vi "Get Wiimote.vi"(8 "error in (no error)":errorcluster, 9 "Wiimote Player #":i32, 11 "LV Wiimote Interface in":T1) -> (0 "error out":errorcluster, 2 "Wiimote":refnum<k24>, 3 "LV Wiimote Interface out":T1)   [LabVIEW 2012, in "LV Wiimote Interface.lvclass"]
uses:
  LV Wiimote Interface.lvclass
  Controls/LV Wiimote Interface.ctl
  C:/Program Files/National Instruments/LabVIEW 2012/vi.lib/LabVIEW Hacker/WiiMote/Dependencies/WiimoteLib.dll
  Program Files/National Instruments/LabVIEW 2012/vi.lib/LabVIEW Hacker/WiiMote/Dependencies/WiimoteLib.dll
  LV Wiimote Interface.lvclass/LV Wiimote Interface.ctl
  <vilib>/Utility/error.llb/Error Cluster From Error Code.vi
  <vilib>/ErrorRing/Error Ring.xnode
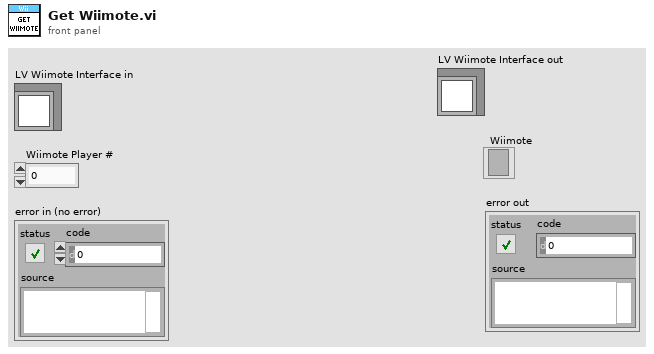
[diagram p1: front panel]
types:
  T1 = typedef "LV Wiimote Interface.ctl" = refnum<class "LV Wiimote Interface.lvclass">
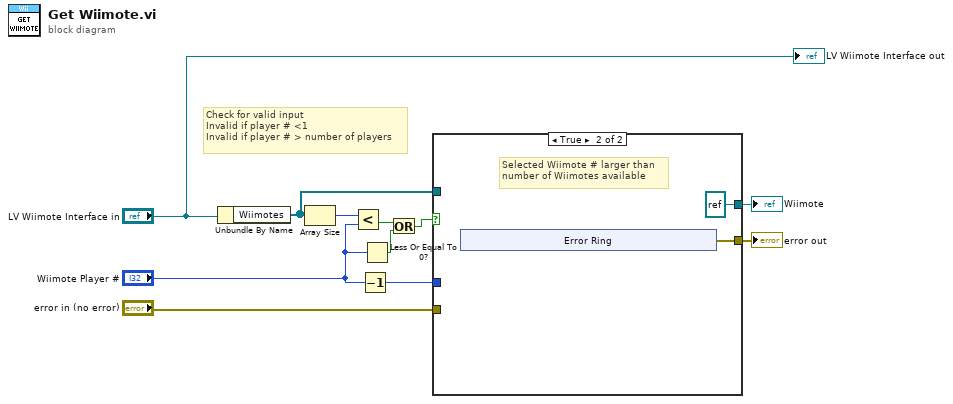
[diagram p0: block diagram]
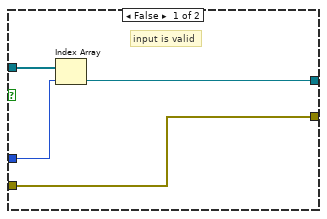
[diagram p2: hidden frame]
diagram:
  # "Check for valid input\nInvalid if player # <1\nInvalid if player # > number of players"
  n1 = Unbundle By Name("LV Wiimote Interface in") -> ("Wiimotes"=w10:refnum<k24>[])
  n2 = Array Size(array=w10) -> (size(s)=w11:i32)
  n3 = Less?(x=w11, y="Wiimote Player #") -> (x < y?=w3:bool)
  n4 = Decrement(x="Wiimote Player #") -> (x-1=w5:i32)
  n5 = Less Or Equal To 0?(x="Wiimote Player #") -> (x <= 0?=w2:bool)
  n6 = Or(x=w3, y=w2) -> (x .or. y?=w1:bool)
  n7 = case shown="True" w1 {
    tunnel: w10 -> [w15 _]
    tunnel: "error in (no error)" -> [w13 _]
    tunnel: [w13 w17] -> w8
    tunnel: [w14 refnum<k24> refnum ("Wiimote")] -> w7
    tunnel: w5 -> [w12 _]
    frame False {
      # "input is valid"
      n8 = Index Array(array=w15, index=w12) -> (element=w14:refnum<k24>)
    }
    frame True {
      # "Selected Wiimote # larger than \nnumber of Wiimotes available"
      n9 = xnode "Error Ring"() -> ("error out"=w17:errorcluster)
    }
  }
  "error out" <- w8
  "Wiimote" <- w7
  "LV Wiimote Interface out" <- "LV Wiimote Interface in"
